vi "dfd_SCL_SOSIIRIITz_CU.vi"(8 "output valid":bool, 9 "global reset":bool) -> (2 "Control signal":T1)   [LabVIEW 2017]
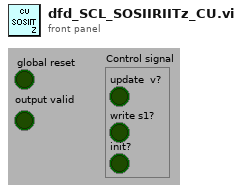
[diagram p1: front panel]
types:
  T1 = cluster{"update  v?":bool, "write s1?":bool, "init?":bool}
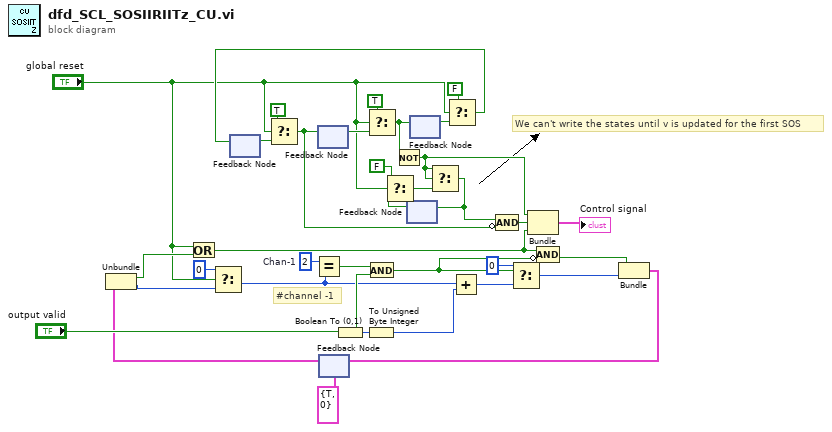
[diagram p0: block diagram]
diagram:
  w28 = u8 2  # Chan-1
  # "We can't write the states until v is updated for the first SOS"
  # "#channel -1"
  n1 = feedback #1() -> (w6:bool)  [unwired: 1 out]
  n2 = Select(t=TRUE, s="global reset", f=w6) -> (s? t:f=w2:bool)
  n3 = feedback-in #2(w2) -> ()
  n4 = feedback #2() -> (w4:bool)  [unwired: 1 out]
  n5 = feedback #3(cluster{"first run?":bool, "Ch cnt":u8} {"first run?"=TRUE, "Ch cnt"=0} ("counter state out")) -> (w24:cluster{"first run?":bool, "Ch cnt":u8})
  n6 = Unbundle(w24) -> ("first run?"=w11:bool, "Ch cnt"=w12:u8)
  n7 = Or(x="global reset", y=w11) -> (x .or. y?=w18:bool)
  n8 = Select(t=u8 0, s="global reset", f=w12) -> (s? t:f=w20:u8)
  n9 = Equal?(x=w28, y=w20) -> (x = y?=w32:bool)
  n10 = Boolean To (0,1)(Boolean="output valid") -> (0, 1=w34:i16)
  n11 = To Unsigned Byte Integer(number=w34) -> (unsigned 8bit integer=w33:u8)
  n12 = Select(t=TRUE, s="global reset", f=w4) -> (s? t:f=w3:bool)
  n13 = And(x=w32, y="output valid") -> (x .and. y?=w26:bool)
  n14 = Not(x=w3) -> (.not. x?=w17:bool)
  n15 = feedback #4() -> (w16:bool)  [unwired: 1 out]
  n16 = Select(t=FALSE, s="global reset", f=w16) -> (s? t:f=w14:bool)
  n17 = feedback-in #5(w3) -> ()
  n18 = feedback #5() -> (w9:bool)  [unwired: 1 out]
  n19 = Select(t=w17, s=w17, f=w14) -> (s? t:f=w13:bool)
  n20 = feedback-in #4(w13) -> ()
  n21 = Select(t=FALSE, s="global reset", f=w9) -> (s? t:f=w8:bool)
  n22 = feedback-in #1(w8) -> ()
  n23 = Add(x=w20, y=w33) -> (x+y=w31:u8)
  n24 = Compound Arithmetic op=AND(w13, invert w2) -> (w22:bool)
  n25 = Select(t=u8 0, s=w26, f=w31) -> (s? t:f=w29:u8)
  n26 = Bundle(w17, w22, w18) -> (→"Control signal":cluster{bool, bool, bool})  [unwired: 1 out]
  n27 = Compound Arithmetic op=AND(w18, invert w26) -> (w19:bool)
  n28 = Bundle(w19, "t"=w29) -> (w23:cluster{bool, "t":u8})  [unwired: 1 out]
  n29 = feedback-in #3(w23) -> ()
